vi "Complete_Controller_part_pressures.vi"() -> ()   [LabVIEW 2014]
uses:
  <vilib>/DAQmx/read.llb/DAQmx Read (Analog 1D DBL NChan 1Samp).vi
  <vilib>/DAQmx/write.llb/DAQmx Write (Analog 1D DBL NChan 1Samp).vi
  <vilib>/DAQmx/write.llb/DAQmx Write (Digital Bool 1Line 1Point).vi
  <vilib>/Instr/_visa.llb/VISA Configure Serial Port (Instr).vi
  <vilib>/Utility/file.llb/Read From Spreadsheet File (string).vi
  <vilib>/DAQmx/miscellaneous.llb/DAQmx Fill In Error Info.vi
  Environmental Chamber LabVIEW and Instruments/Drivers and Software/keithley_6430/Keithley 6430/Public/Data/Read (Single Point).vi
  Environmental Chamber LabVIEW and Instruments/Drivers and Software/LabVIEW 8.2 Drivers/keithley_24xx/Keithley 24XX/Public/Data/Read (Single Point).vi
  <vilib>/Utility/file.llb/Write To Spreadsheet File (string).vi
  Environmental Chamber LabVIEW and Instruments/Drivers and Software/keithley_24xx/Keithley 24XX/Keithley 24XX.lvlib
  Environmental Chamber LabVIEW and Instruments/Drivers and Software/keithley_6430/Keithley 6430/Keithley 6430.lvlib
panel:
  in  "Turbo pump\nauto on":bool=TRUE
  in  "Use excel file\nfor sequence?":bool
  out "Sequence time left (hrs)":dbl caption="min"
  out "Sequence Preview":cluster{dbl[], dbl[]}[](graph)
  in  "Import sequence file":path
  out "Chamber relative humidity (%)":dbl
  out "Pressure Control 3":bool caption="Pressure Control"
  in  "valve % open":dbl=100.0 min=0.0 max=100.0 step=5.0
  out "Pressure Control 2":bool caption="Pressure Control"
  out "Keithley 6430":bool
  out "J-Kem":bool caption="J-Kem Temp"
  out "Thermometer":dbl(slide) scale=0.0..150.0
  out "J-Kem Temp (C)":cluster{dbl}(graph)
  out "Keithley 2420":bool caption="Keithley 2430"
  out "Pressure Control":bool
  out "Arduino":bool
  out "SRS QCM":bool
  out "Chamber Pressure (Torr)":cluster{"f":dbl}(graph)
  in  "Start recording after":dbl caption="min"
  in  "Auto stop after":bool
  in  "hrs":dbl=1000.0 min=0.0
  out "Start Time":string
  out "Elapsed (min)":dbl caption="Elapsed Time (s)"
  in  "Delay between data points (s)":dbl caption="sec" min=0.0 max=30.0 format="%#_13g"
  in  "Vapor\nflow\n(sccm)":sgl(slide) min=0 max=100 step=1 scale=0.0..100.0
  out "Actual":dbl
  out "Boolean 3":bool
  out "Actual":dbl
  out "Boolean":bool
  in  "Gas\nflow\n(sccm)":sgl(slide) min=0 max=100 step=1 scale=0.0..100.0
  in  "Turbo pump auto on":bool
  in  "Desired pressure":dbl min=0.0 max=760.0 step=5.0
  out "Valve position (%)":dbl
  in  "Pressure Control":enum32{"Open Mode (%)", "Pressure Mode (Torr)"}(radio)
  in  "stop":bool
  in  "Experiment Notes":string
  in  "Clear all charts":bool
  out "Save data file path":path
  out "Waveform Chart 2":cluster{"f":dbl, "f":dbl}(graph)
  out "Keithley 2420 (Ohm)":cluster{"Resistance":sgl}(graph)
  out "Keithley 6430 (Ohm)":cluster{"Measurement":dbl}(graph)
  out "temp\n(C)":string
  out "gas\nsensor":string
  out "Arduino humidity (%)":cluster{dbl}(graph)
  out "MHz":dbl format="%.6f"
  out "Ohm":dbl format="%.4e"
  out "Waveform Chart 7":cluster{dbl, "Resistance out":dbl}(graph)
  in  "Tab Control":enum32{"Run Sequence", "Create Sequence"}(tab)
  out "User-defined\nsequence 2":string[][](table) caption="Sequence to run"
  in  "Run Sequence":bool
  out "Current step":i32
  out "Step time remaining (min)":dbl caption="min"
  in  "User-defined\nsequence":string[][](table) caption="Create sequence"
  out "QCM mass deposited (g)":cluster{dbl}(graph)
  in  "rapidox O2 Sensor":bool
  in  "setnag O2 Pump":bool
  in  "Baud Rate 2":i32(ring)=2 items=["2400", "4800", "9600", "19200", "38400", "57600", "115200"]
  in  "Com Port":i32(ring) items=["Com 1", "Com 2", "Com 3", "Com 4", "Com 5", "Com 6", "COM 7", "COM 8", "COM 9", "COM 10", "COM 11", "COM 12", "com 13", "COM 14"]
  in  "Com Port 2":i32(ring) items=["Com 1", "Com 2", "Com 3", "Com 4", "Com 5", "Com 6", "COM 7", "COM 8", "COM 9", "COM 10", "COM 11", "COM 12", "com 13", "COM 14"]
  out "Torr":dbl
  out "%":dbl
  out "atm":dbl
  out "Waveform Chart":cluster{dbl}(graph)
  out "O2 Concentration (PPM)":dbl
  out "Waveform Chart 6":cluster{dbl}(graph)
  # "Sample\ntemp (C)"
  # "Currently Unused"
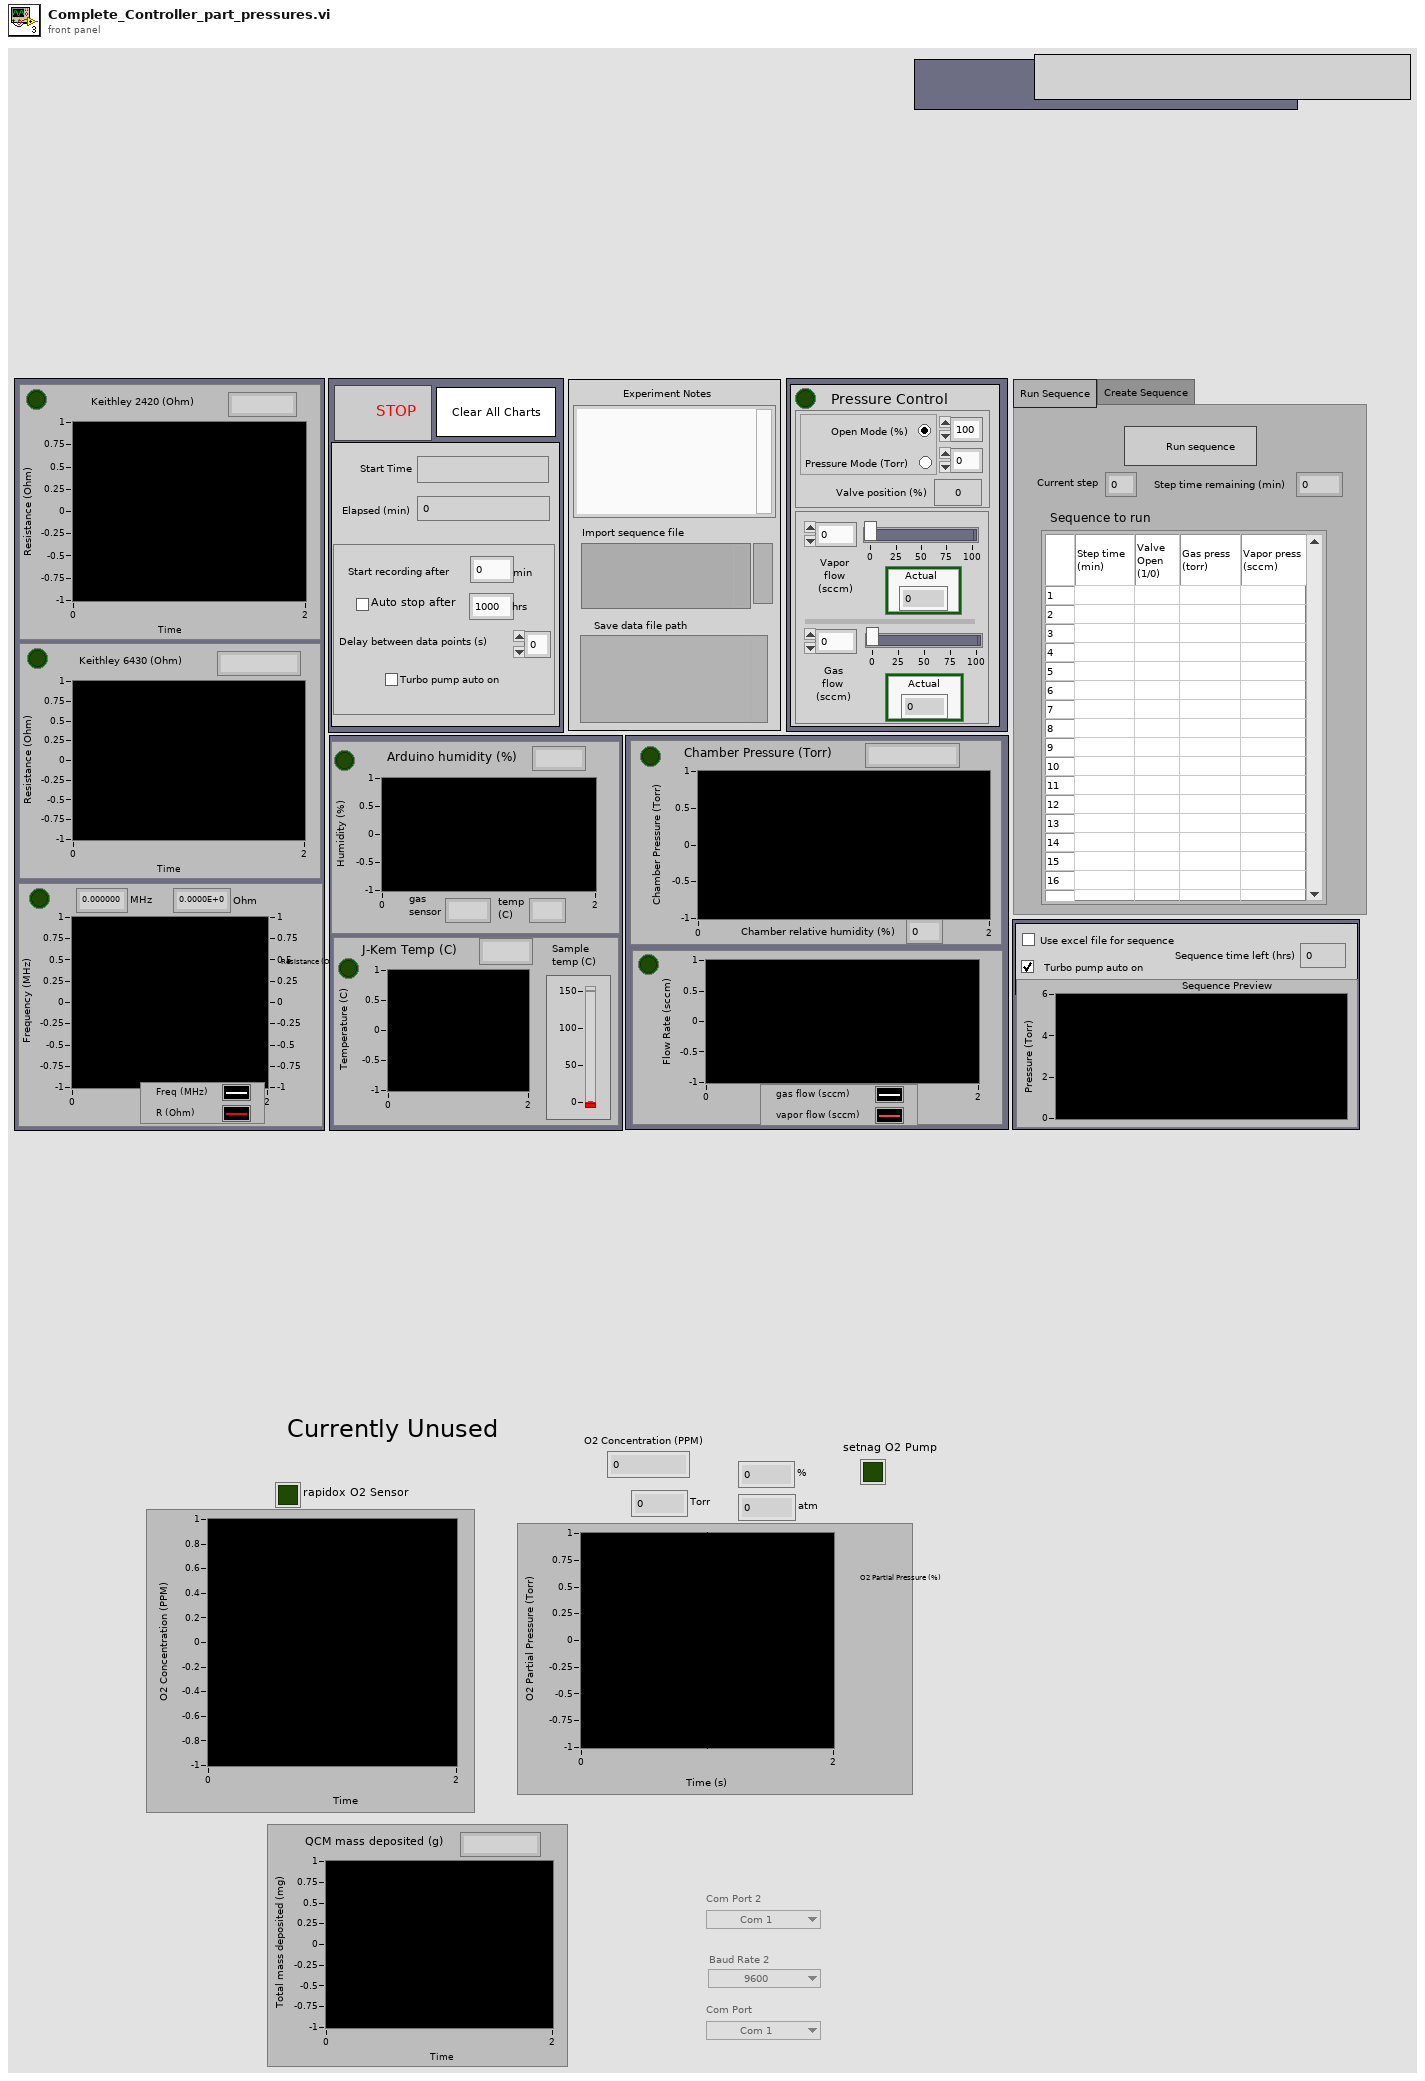
[diagram p1: front panel]
types:
  T1 = enum16{"open", "open or create", "create or replace", "create", "open (read only)"}
  T2 = enum16{"no parity", "odd parity", "even parity", "mark parity", "space parity"}
  T3 = cluster{bool, "VISA resource name":refnum<visa-resource-name>, "error out":errorcluster}
  T4 = cluster{bool, "VISA resource name out":refnum<visa-resource-name>, "error out":errorcluster}
  T5 = cluster{"task out":refnum<k21>, "error out":errorcluster, "task out":refnum<k21>, "error out":errorcluster, "task out":refnum<k21>, "error out":errorcluster, "VISA resource name":refnum<visa-resource-name>, "error out":errorcluster}
  T6 = cluster{"task out":refnum<k21>, "error out":errorcluster, "task out":refnum<k21>, "error out":errorcluster, "task out":refnum<k21>, "error out":errorcluster, "VISA resource name out":refnum<visa-resource-name>, "error out":errorcluster}
  T7 = cluster{bool, "VISA out":refnum<visa-resource-name>, "error out":errorcluster}
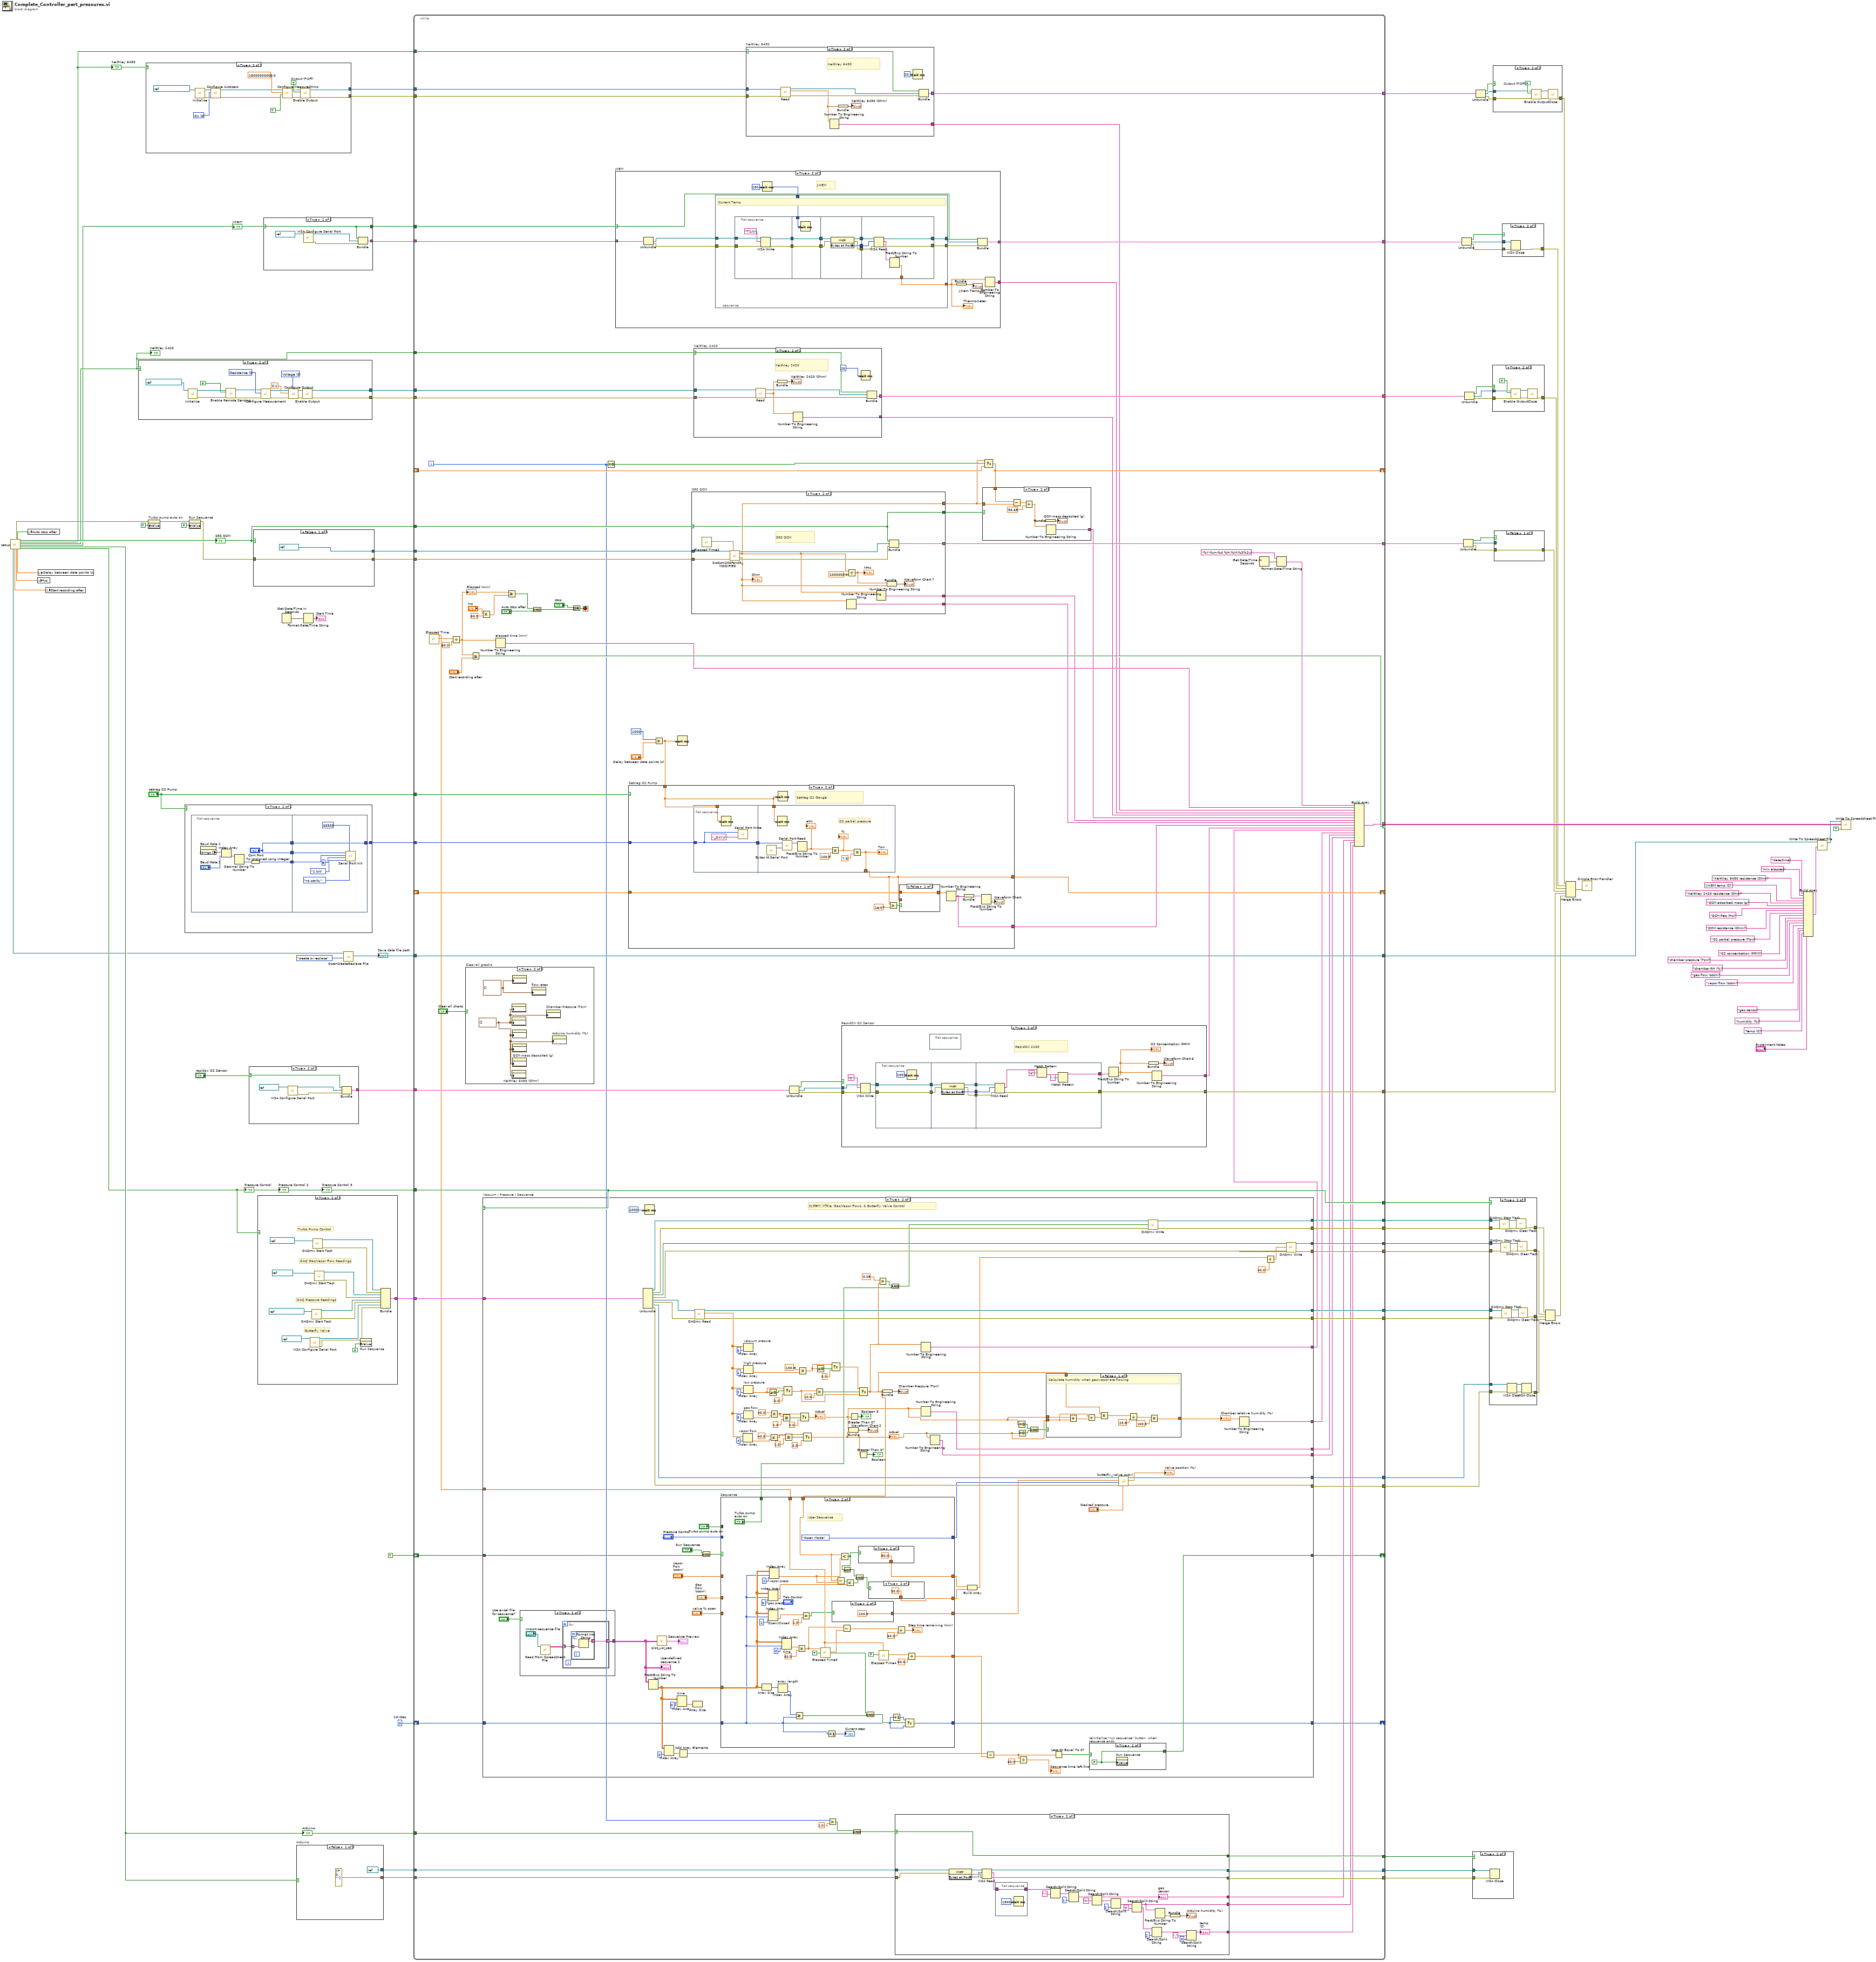
[diagram p0: block diagram]
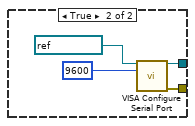
[diagram p3: hidden frame]
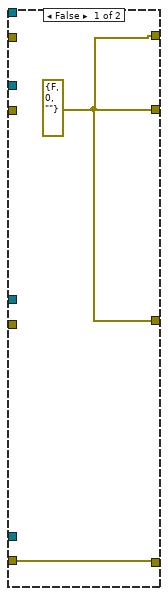
[diagram p4: hidden frame]
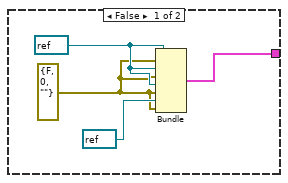
[diagram p5: hidden frame]
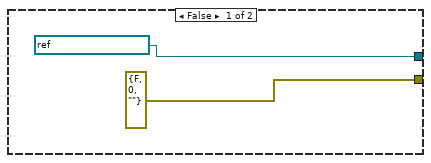
[diagram p7: hidden frame]
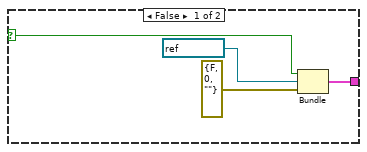
[diagram p8: hidden frame]
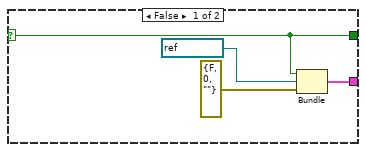
[diagram p10: hidden frame]
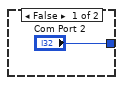
[diagram p11: hidden frame]
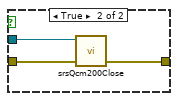
[diagram p12: hidden frame]
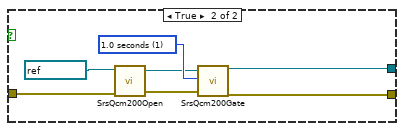
[diagram p13: hidden frame]
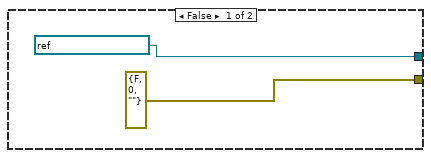
[diagram p15: hidden frame]
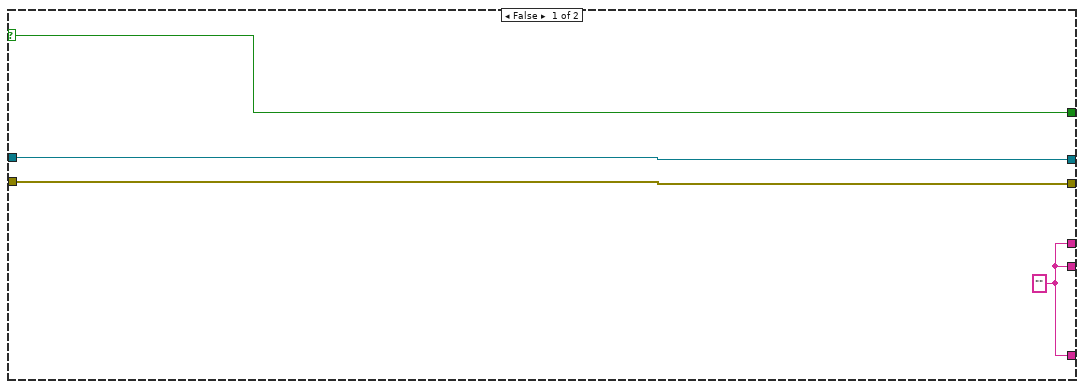
[diagram p16: hidden frame]
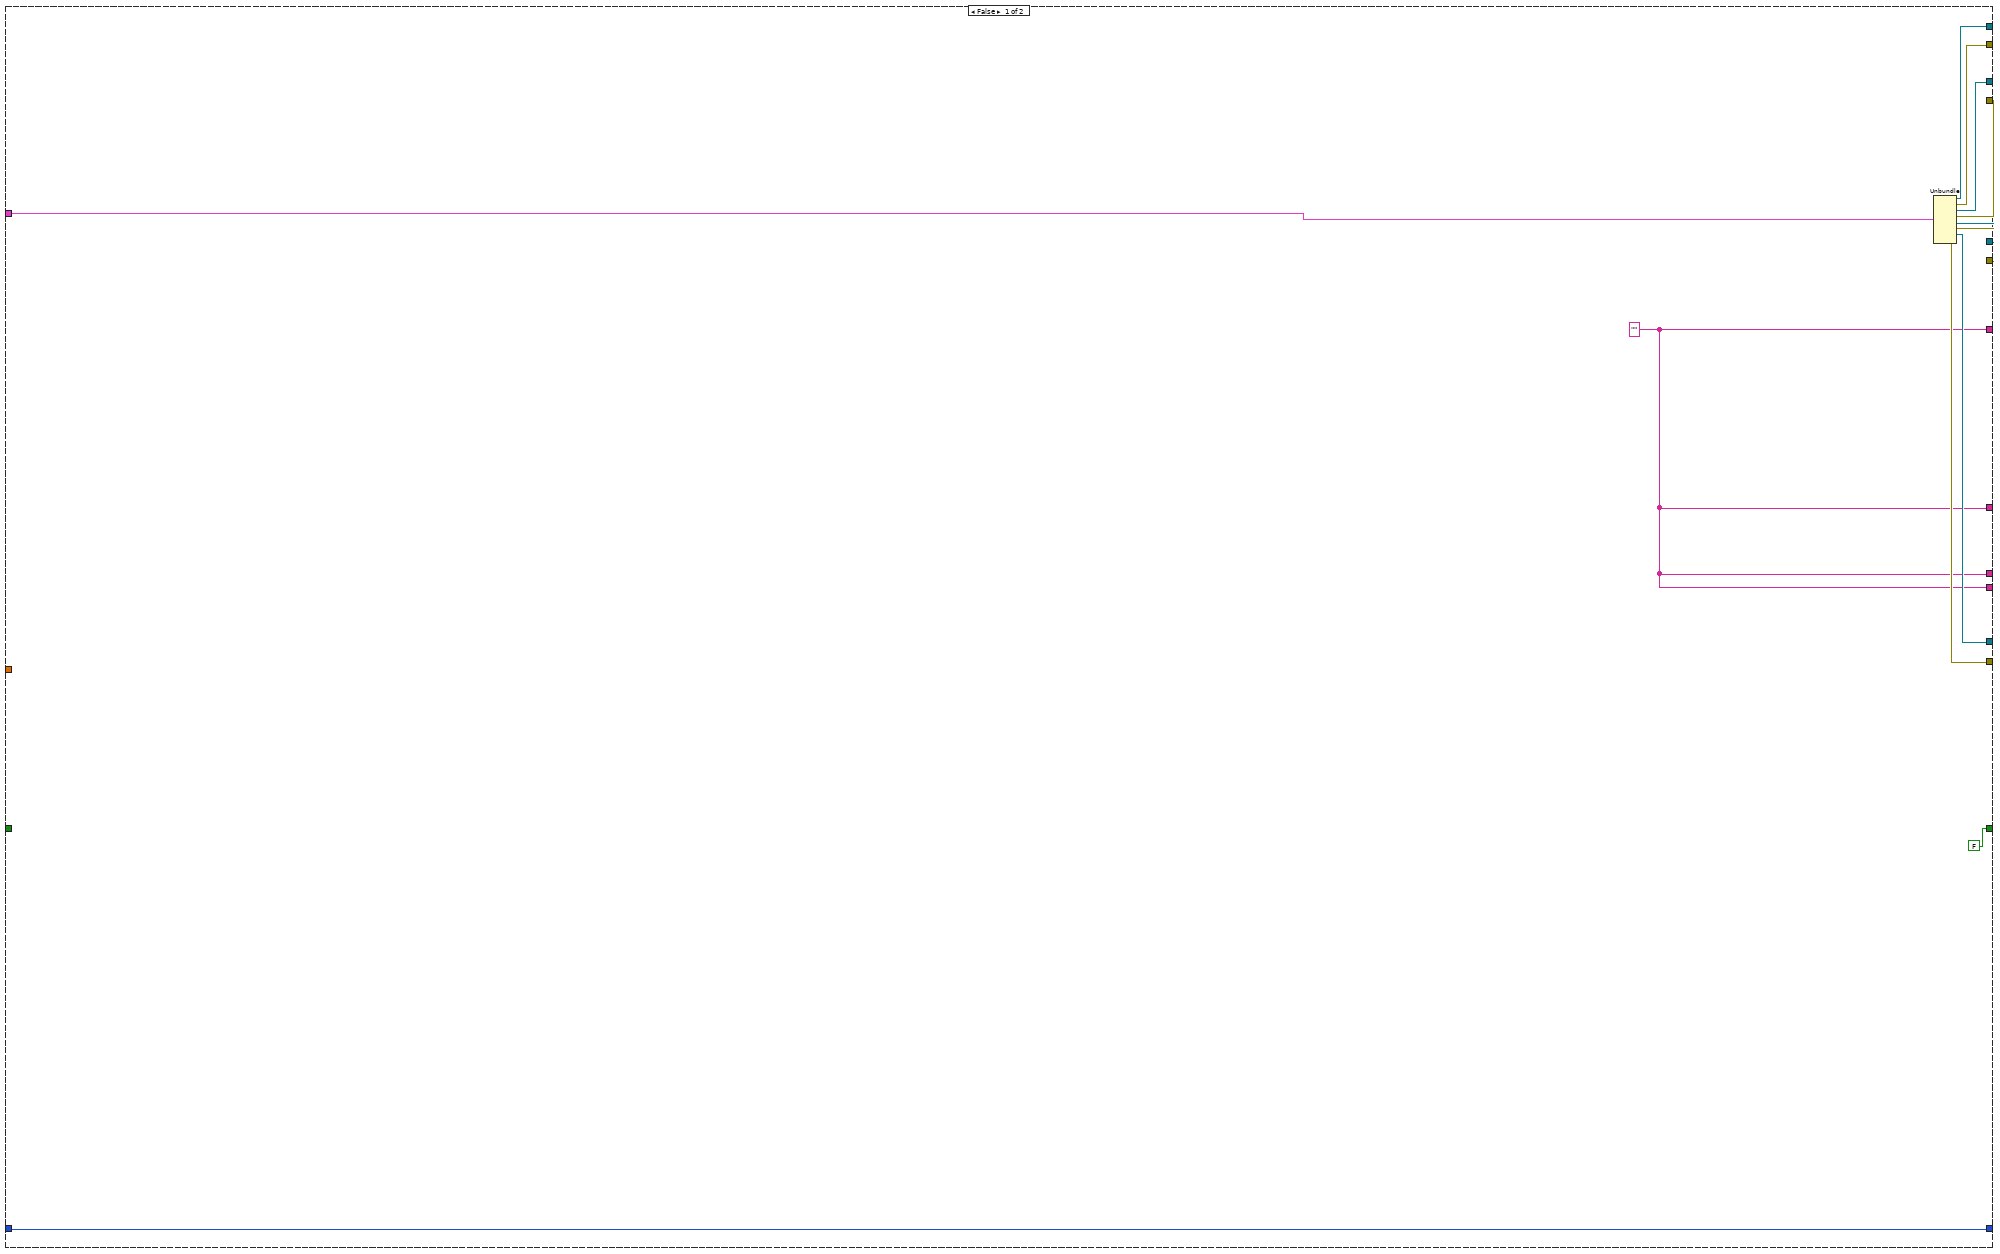
[diagram p17: hidden frame]
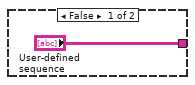
[diagram p18: hidden frame]
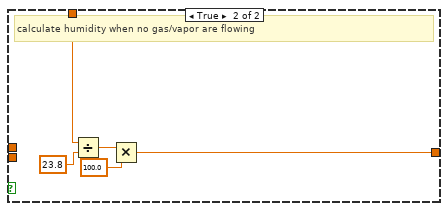
[diagram p19: hidden frame]
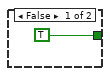
[diagram p20: hidden frame]
diagram:
  w29 = 0  # 1st step
  n1 = call "setup.vi"() -> ("Save file path 2"=w10:path, "begin recording"=w16:dbl, "error IO"=w3:errorcluster, "stop after"=w18:dbl, "Auto Stop 2"=w19:bool, "delay 5"=w17:dbl, "SRS QCM 2"=w15:bool, "Keithley 6431"=w11:bool, "Keithley 2421"=w14:bool, "J-KEM2"=w13:bool, "Arduino2"=w12:bool, "Pressure control 2"=w9:bool)  [unwired: 8 in]
  "SRS QCM" <- w15
  "Arduino" <- w12
  "Pressure Control" <- w9
  "Keithley 2420" <- w14
  "J-Kem" <- w13
  "Keithley 6430" <- w11
  "Pressure Control 2" <- w9
  "Pressure Control 3" <- w9
  n2 = local write "Auto stop after"(w19) -> ()
  n3 = local write "hrs"(w18) -> ()
  n4 = local write "Delay between data points (s)"(w17) -> ()
  n5 = local write "Start recording after"(w16) -> ()
  n6 = case shown="True" w14 {
    tunnel: [refnum<visa-resource-name> "GPIB1::24::INSTR" ("VISA resource name") w108] -> w96
    tunnel: [errorcluster {"status"=FALSE, "code"=0, "source"=""} ("error out") w103] -> w95
    frame False {
    }
    frame True {
      w110 = u16 0 items=["Voltage", "Current"] ("Source Mode  (0: Voltage)")
      w115 = u16 2 items=["Volts", "Current", "Resistance"] ("Function (0: Volts)")
      n7 = call "Initialize.vi"("VISA resource name"=refnum<visa-resource-name> "GPIB1::24::INSTR") -> ("error out"=w104:errorcluster, "VISA resource name out"=w107:refnum<visa-resource-name>)  [unwired: 9 in]
      n8 = call "Enable Remote Sensing.vi"("error in (no error)"=w104, "Enable Remote Sensing (T: Enable)"=FALSE ("4-wire?"), "VISA resource name"=w107) -> ("error out"=w105:errorcluster, "VISA resource name out"=w106:refnum<visa-resource-name>)  [unwired: 7 in]
      n9 = call "Configure Measurement.vi"("error in (no error)"=w105, "Function (0: Volts)"=w115, "VISA resource name"=w106) -> ("error out"=w114:errorcluster, "VISA resource name out"=w113:refnum<visa-resource-name>)  [unwired: 7 in]
      n10 = call "Configure Output.vi"("Source Mode  (0: Voltage)"=w110, "error in (no error)"=w114, "Output Level (0)"=0.1 ("Applied Voltage (V)"), "VISA resource name"=w113) -> ("error out"=w112:errorcluster, "VISA resource name out"=w111:refnum<visa-resource-name>)  [unwired: 6 in]
      n11 = call "Enable Output.vi"("error in (no error)"=w112, "VISA resource name"=w111) -> ("error out"=w103:errorcluster, "VISA resource name out"=w108:refnum<visa-resource-name>)  [unwired: 8 in]
    }
  }
  n12 = case shown="True" w11 {
    tunnel: [refnum<visa-resource-name> "GPIB0::29::INSTR" ("VISA resource name") w126] -> w53
    tunnel: [errorcluster {"status"=FALSE, "code"=0, "source"=""} ("error out") w127] -> w52
    frame False {
    }
    frame True {
      w122 = u16 0 items=["On", "Off", "Once"] ("Autozero  (0: On)")
      w130 = TRUE  # Output (F:Off)
      n13 = call "Initialize.vi"("VISA resource name"=refnum<visa-resource-name> "GPIB0::29::INSTR") -> ("error out"=w123:errorcluster, "VISA resource name out"=w124:refnum<visa-resource-name>)  [unwired: 4 in, 5 out]
      n14 = call "Configure Autozero.vi"("error in (no error)"=w123, "Autozero  (0: On)"=w122, "VISA resource name"=w124) -> ("error out"=w119:errorcluster, "VISA resource name out"=w120:refnum<visa-resource-name>)  [unwired: 7 in]
      n15 = call "Configure MeasureOhms.vi"("error in (no error)"=w119, "Auto Range (T:Enable)"=TRUE, "Resistance Range [Ohms]"=15000000000.0, "VISA resource name"=w120) -> ("error out"=w131:errorcluster, "VISA resource name out"=w129:refnum<visa-resource-name>)  [unwired: 2 in, 4 out]
      n16 = call "Enable Output.vi"("error in (no error)"=w131, "Enable Output (F:Off)"=w130, "VISA resource name"=w129) -> ("error out"=w127:errorcluster, "VISA resource name out"=w126:refnum<visa-resource-name>)  [unwired: 7 out]
    }
  }
  n17 = property on="Turbo pump auto on" class="Bool (strict)"(error in=w3, "Value"=TRUE ("Turbo\npump")) -> (error out=w2:errorcluster)  [unwired: 1 in, 1 out]
  n18 = case shown="True" "setnag O2 Pump" {
    tunnel: ["Com Port 2" w133] -> w92
    frame False {
    }
    frame True {
      n19 = flat-sequence {
        tunnel: ["Com Port"] -> w136
        tunnel: [w138] -> w135
        tunnel: ["Com Port"] -> w134
        tunnel: w136 -> [w144]
        tunnel: w135 -> [w143]
        tunnel: w134 -> [w145]
        tunnel: [w145] -> w133
        frame #0 {
          n20 = property on="Baud Rate 2" class="Ring (strict)"() -> ("Strings []"=w140:string[])  [unwired: 2 in, 2 out]
          n21 = Index Array(array=w140, index="Baud Rate 2") -> (element=w141:string)
          n22 = Decimal String To Number(string=w141) -> (number=w139:i32)  [unwired: 2 in, 1 out]
          n23 = To Unsigned Long Integer(number=w139) -> (unsigned 32bit integer=w138:u32)
        }
        frame #1 {
          n24 = call <vilib>:"Serial Port Init.vi"("parity"=T2."no parity", "buffer size"=u16 65535, "stop bits"=enum16{"1 bit", "1.5 bits", "2 bits"}."1 bit", "data bits"=u16 8, "baud rate"=w143, "port number"=w144) -> ()  [unwired: 1 in, 1 out]
        }
      }
    }
  }
  n25 = property on="Run Sequence" class="Bool (strict)"(error in=w2, "Value"=FALSE ("Run Sequence")) -> (error out=w7:errorcluster)  [unwired: 1 in, 1 out]
  n26 = case shown="True" "rapidox O2 Sensor" {
    selector: "rapidox O2 Sensor" -> [w150 w155]
    tunnel: [w151 w156] -> w63
    frame False {
      n27 = Bundle(w150, "VISA resource name"=refnum<visa-resource-name> "COM7", "error out"=errorcluster {"status"=FALSE, "code"=0, "source"=""}) -> (w151:T3)  [unwired: 1 in]
    }
    frame True {
      n28 = call-poly "VISA Configure Serial Port"("VISA resource name"=refnum<visa-resource-name> "COM7") -> ("VISA resource name out"=w157:refnum<visa-resource-name>, "error out"=w154:errorcluster)  [unwired: 13 in]
      n29 = Bundle(w155, "VISA resource name out"=w157, "error out"=w154) -> (w156:T4)  [unwired: 1 in]
    }
  }
  n30 = case shown="False" w15 {
    tunnel: [refnum<visa-resource-name> "COM6" ("VISA in") w163] -> w94
    tunnel: [w159 w162] -> w93
    tunnel: w7 -> [w159 w161]
    frame False {
    }
    frame True {
      w167 = u16 1 items=["0.1 seconds", "1.0 seconds", "10.0 seconds"] ("Gate in")
      n31 = call "SrsQcm200Open.vi"("error in"=w161, "VISA in"=refnum<visa-resource-name> "COM6") -> ("error out"=w164:errorcluster, "VISA out"=w165:refnum<visa-resource-name>)  [unwired: 3 in]
      n32 = call "SrsQcm200Gate.vi"("VISA in"=w165, "Gate in"=w167, "error in (no error)"=w164) -> ("VISA out"=w163:refnum<visa-resource-name>, "error out"=w162:errorcluster)  [unwired: 14 in, 1 out]
    }
  }
  n33 = case shown="True" w9 {
    tunnel: [w168 w175] -> w34
    frame False {
      w170 = refnum<k21> refnum ("task out")
      w169 = errorcluster {"status"=FALSE, "code"=0, "source"=""} ("error out")
      n34 = Bundle("task out"=w170, "error out"=w169, "task out"=w170, "error out"=w169, "task out"=w170, "error out"=w169, "VISA resource name"=refnum<visa-resource-name> refnum, "error out"=w169) -> (w168:T5)  [unwired: 1 in]
    }
    frame True {
      # "Turbo Pump Control"
      # "DAQ Gas/Vapor Flow Readings"
      # "DAQ Pressure Readings"
      # "Butterfly Valve"
      n35 = call-poly "VISA Configure Serial Port"("VISA resource name"=refnum<visa-resource-name> "COM5") -> ("VISA resource name out"=w176:refnum<visa-resource-name>, "error out"=w172:errorcluster)  [unwired: 13 in]
      n36 = call <vilib>:"DAQmx Start Task.vi"("task/channels in"=refnum<k21> "AllDaqReadings") -> ("task out"=w178:refnum<k21>, "error out"=w177:errorcluster)  [unwired: 13 in]
      n37 = call <vilib>:"DAQmx Start Task.vi"("task/channels in"=refnum<k21> "TurboON") -> ("task out"=w182:refnum<k21>, "error out"=w181:errorcluster)  [unwired: 13 in]
      n38 = call <vilib>:"DAQmx Start Task.vi"("task/channels in"=refnum<k21> "Setflow") -> ("task out"=w180:refnum<k21>, "error out"=w179:errorcluster)  [unwired: 13 in]
      n39 = property on="Run Sequence" class="Bool (strict)"(error in=w172, "Value"=FALSE ("Run Sequence")) -> (error out=w174:errorcluster)  [unwired: 1 in, 1 out]
      n40 = Bundle("task out"=w182, "error out"=w181, "task out"=w180, "error out"=w179, "task out"=w178, "error out"=w177, "VISA resource name out"=w176, "error out"=w174) -> (w175:T6)  [unwired: 1 in]
    }
  }
  n41 = case shown="True" w13 {
    selector: w13 -> [w187 w192]
    tunnel: [w188 w193] -> w81
    tunnel: [w187 w192] -> w75
    frame False {
      n42 = Bundle(w187, "VISA resource name"=refnum<visa-resource-name> "COM3", "error out"=errorcluster {"status"=FALSE, "code"=0, "source"=""}) -> (w188:T3)  [unwired: 1 in]
    }
    frame True {
      n43 = call-poly "VISA Configure Serial Port"("VISA resource name"=refnum<visa-resource-name> "COM3") -> ("VISA resource name out"=w194:refnum<visa-resource-name>, "error out"=w191:errorcluster)  [unwired: 13 in]
      n44 = Bundle(w192, "VISA resource name out"=w194, "error out"=w191) -> (w193:T4)  [unwired: 1 in]
    }
  }
  n45 = Get Date/Time In Seconds() -> (seconds since 1Jan1904=w99:timestamp)
  n46 = case "Arduino" shown="False" w12 {
    tunnel: [refnum<visa-resource-name> refnum ("VISA resource name out") w201] -> w28
    tunnel: [errorcluster {"status"=FALSE, "code"=0, "source"=""} ("error out") w198] -> w27
    frame False {
    }
    frame True {
      n47 = call-poly "VISA Configure Serial Port"("VISA resource name"=refnum<visa-resource-name> "COM12", "baud rate (9600)"=u32 9600) -> ("VISA resource name out"=w201:refnum<visa-resource-name>, "error out"=w198:errorcluster)  [unwired: 12 in]
    }
  }
  n48 = Format Date/Time String(seconds (now)=w99) -> (date/time string=→"Start Time":string)  [unwired: 2 in]
  n49 = call "OpenCreateReplace File.vi"("function (open:0)"=T1."create or replace", "file path"=w10) -> ("new file path"=w20:path)  [unwired: 6 in, 3 out]
  "Save data file path" <- w20
  n50 = while {
    shift-right: [w291] -> _
    shift-left: _ -> [w290]
    tunnel: [w220] -> w97 mode=indexing if=w219
    tunnel: w14 -> [w259]
    tunnel: w96 -> [w288]
    tunnel: w95 -> [w287]
    tunnel: w94 -> [w286]
    tunnel: w93 -> [w285]
    tunnel: w15 -> [w283]
    tunnel: "setnag O2 Pump" -> [w276]
    tunnel: w92 -> [w282]
    tunnel: [w278] -> w89
    tunnel: [w277] -> w85
    tunnel: w81 -> [w275]
    tunnel: [w274] -> w80
    tunnel: w75 -> [w272]
    tunnel: w63 -> [w268]
    tunnel: [w263] -> w61
    tunnel: [w258] -> w60
    tunnel: w20 -> [w258]
    shift-right: [w241] -> _
    shift-left: _ -> [w243]
    tunnel: w53 -> [w255]
    tunnel: w52 -> [w254]
    tunnel: [w253] -> w51
    tunnel: w11 -> [w252]
    tunnel: w9 -> [w233]
    tunnel: [w249] -> w47
    tunnel: [w248] -> w44
    tunnel: [w247] -> w46
    tunnel: [w246] -> w45
    tunnel: [w233] -> w43
    tunnel: [w245] -> w38
    tunnel: w34 -> [w237]
    tunnel: [w236] -> w32
    tunnel: [w235] -> w31
    tunnel: [w234] -> w30
    shift-right: [w232] -> _
    shift-left: w29 -> [w231]
    tunnel: w12 -> [w216]
    tunnel: w28 -> [w226]
    tunnel: w27 -> [w225]
    tunnel: [w224] -> w26
    tunnel: [w223] -> w25
    tunnel: [w222] -> w24
    shift-right: [w207] -> _
    shift-left: TRUE -> [w208]
    i -> [w205]
    stop <- w271 stop-if-true
    n51 = call "Elapsed Time"() -> ("Present (s)"=w230:dbl, "Elapsed Time (s)"=w270:dbl)  [unwired: 12 in, 6 out]
    n52 = Divide(x=w270, y=60.0) -> (x/y=w210:dbl)
    "Elapsed (min)" <- w210
    n53 = case "Clear all graphs" shown="True" "Clear all charts" {
      frame False {
      }
      frame True {
        w547 = cluster{dbl, "Resistance out":dbl}[] [] ("History Data")
        w546 = cluster{dbl}[] [] ("History Data")
        n54 = property on="Keithley 2420 (Ohm)" class="WFChart (strict)"("History Data"=w546) -> ()  [unwired: 2 in, 2 out]
        n55 = property on="J-Kem Temp (C)" class="WFChart (strict)"("History Data"=w546) -> ()  [unwired: 2 in, 2 out]
        n56 = property on="Keithley 6430 (Ohm)" class="WFChart (strict)"("History Data"=w546) -> ()  [unwired: 2 in, 2 out]
        n57 = property on="Waveform Chart 7" class="WFChart (strict)"("History Data"=w547) -> ()  [unwired: 2 in, 2 out]
        n58 = property on="Waveform Chart" class="WFChart (strict)"("History Data"=w546) -> ()  [unwired: 2 in, 2 out]
        n59 = property on="Waveform Chart 6" class="WFChart (strict)"("History Data"=w546) -> ()  [unwired: 2 in, 2 out]
        n60 = property on="QCM mass deposited (g)" class="WFChart (strict)"("History Data"=w546) -> ()  [unwired: 2 in, 2 out]
        n61 = property on="flow rates" class="WFChart (strict)"("History Data"=w547) -> ()  [unwired: 2 in, 2 out]
        n62 = property on="Chamber Pressure (Torr)" class="WFChart (strict)"("History Data"=w546) -> ()  [unwired: 2 in, 2 out]
        n63 = property on="Arduino humidity (%)" class="WFChart (strict)"("History Data"=w546) -> ()  [unwired: 2 in, 2 out]
      }
    }
    n64 = Greater Or Equal?(x=w210, y="Start recording after") -> (x >= y?=w219:bool)
    n65 = Multiply(x="hrs", y=60.0) -> (x*y=w202:dbl)
    n66 = case "Vacuum / Pressure / Sequence" shown="True" w233 {
      tunnel: [w333 w440] -> w248
      tunnel: [w334 w439] -> w246
      tunnel: [w336 w420] -> w249
      tunnel: [w335 w421] -> w247
      tunnel: [w334 w411] -> w245
      tunnel: [w329 w401] -> w240
      tunnel: [w329 w400] -> w239
      tunnel: [w329 w398] -> w238
      tunnel: w237 -> [w339 w396]
      tunnel: [w338 w387] -> w236
      tunnel: [w337 w386] -> w235
      tunnel: [w332 w385] -> w234
      tunnel: w231 -> [w331 w368]
      tunnel: [w331 w382] -> w232
      tunnel: w230 -> [_ w381]
      tunnel: w208 -> [_ w361]
      tunnel: [FALSE ("new element/subarray") w356] -> w207
      tunnel: [w329 w355] -> w206
      frame False {
        w329 = ""
        n67 = Unbundle(w339) -> ("task out"=w338:refnum<k21>, "error out"=w337:errorcluster, "task out"=w336:refnum<k21>, "error out"=w335:errorcluster, "task out"=w333:refnum<k21>, "error out"=w334:errorcluster, "VISA resource name out"=w332:refnum<visa-resource-name>)  [unwired: 1 out]
      }
      frame True {
        # "system info"
        # "DAQ Pressure, Gas/Vapor Flows, & Butterfly Valve Control"
        n68 = case shown="True" "Use excel file\nfor sequence?" {
          tunnel: ["User-defined\nsequence" w443] -> w348
          frame False {
          }
          frame True {
            n69 = call-poly <vilib>:"Read From Spreadsheet File.vi"("file path (dialog if empty)"="Import sequence file") -> ("all rows"=w445:string[][])  [unwired: 6 in, 4 out]
            n70 = for {
              tunnel: w445 -> [w447] mode=indexing
              tunnel: [w446] -> w443 mode=indexing
              n71 = for {
                tunnel: w447 -> [w449] mode=indexing
                tunnel: [w448] -> w446 mode=indexing
                n72 = Format Into String(w449) -> (resulting string=w448:string)  [unwired: 3 in, 1 out]
              }
            }
          }
        }
        "User-defined\nsequence 2" <- w348
        n73 = Unbundle(w396) -> ("task out"=w389:refnum<k21>, "error out"=w388:errorcluster, "task out"=w390:refnum<k21>, "error out"=w391:errorcluster, "task out"=w392:refnum<k21>, "error out"=w393:errorcluster, "VISA resource name out"=w394:refnum<visa-resource-name>, "error out"=w395:errorcluster)
        n74 = Wait (ms)(milliseconds to wait=u32 1000) -> ()  [unwired: 1 out]
        n75 = Fract/Exp String To Number(string=w348) -> (number=w360:dbl[][])  [unwired: 3 in, 1 out]
        n76 = call "plot_usr_seq.vi"("User-defined sequence"=w348) -> ("Sequence Preview"=→"Sequence Preview":cluster{dbl[], dbl[]}[])
        n77 = Index Array(array=w360, index (col)=0 ("disabled index (col)")) -> (element=w372:dbl[])  [unwired: 1 in]
        n78 = Index Array "time"(array=w360, index (row)=0 ("disabled index (col)")) -> (element=w359:dbl[])  [unwired: 1 in]
        n79 = Add Array Elements(numeric array=w372) -> (sum=w365:dbl)
        n80 = Array Size(array=w359) -> ()  [unwired: 1 out]
        n81 = call-poly <vilib>:"DAQmx Read.vi"("task/channels in"=w392, "error in"=w393) -> ("task out"=w440:refnum<k21>, "data"=w431:dbl[], "error out"=w439:errorcluster)  [unwired: 11 in]
        n82 = And(x="Run Sequence", y=w361) -> (x .and. y?=w362:bool)
        n83 = Index Array "vapor flow"(array=w431, index=4) -> (element=w427:dbl)
        n84 = Index Array "vacuum presure"(array=w431, index=0) -> ()  [unwired: 1 out]
        n85 = Index Array "high pressure"(array=w431, index=1) -> (element=w434:dbl)
        n86 = Index Array "low pressure"(array=w431, index=2) -> (element=w405:dbl)
        n87 = Index Array "gas flow"(array=w431, index=3) -> (element=w429:dbl)
        n88 = Greater Or Equal To 0?(x=w405) -> (x >= 0?=w406:bool)
        n89 = Multiply(x=40.0, y=w427) -> (x*y=w418:dbl)
        n90 = Multiply(x=40.0, y=w429) -> (x*y=w415:dbl)
        n91 = Greater Or Equal?(x=w415, y=1.0) -> (x >= y?=w414:bool)
        n92 = Select(t=w405, s=w406, f=0.0) -> (s? t:f=w404:dbl)
        n93 = Greater Or Equal?(x=w418, y=1.0) -> (x >= y?=w417:bool)
        n94 = Multiply(x=100.0, y=w434) -> (x*y=w422:dbl)
        n95 = Select(t=w415, s=w414, f=0.0) -> (s? t:f=w350:dbl)
        "Actual" <- w350
        n96 = Select(t=w418, s=w417, f=0.0) -> (s? t:f=w349:dbl)
        "Actual" <- w349
        n97 = Greater?(x=w404, y=10.0) -> (0:w410:bool)
        n98 = Greater Or Equal To 0?(x=w422) -> (x >= 0?=w424:bool)
        n99 = Select(t=w422, s=w424, f=0.0) -> (s? t:f=w409:dbl)
        n100 = Bundle("f"=w350, "f"=w349) -> (→"Waveform Chart 2":cluster{"f":dbl, "f":dbl})  [unwired: 1 in]
        n101 = Greater Than 0?(x=w350) -> (x > 0?=→"Boolean 3":bool)
        n102 = Select(t=w409, s=w410, f=w404) -> (s? t:f=w340:dbl)
        n103 = case "Sequence" shown="True" w362 {
          tunnel: w381 -> [_ w502]
          tunnel: [w473 w503] -> w382
          tunnel: w368 -> [w473 w489]
          tunnel: "Vapor\nflow\n(sccm)" -> [w472 _]
          tunnel: "Gas\nflow\n(sccm)" -> [w471 _]
          tunnel: [w472 w483] -> w378
          tunnel: [w471 w474] -> w377
          tunnel: "Turbo pump auto on" -> [w470 _]
          tunnel: [w470 "Turbo pump\nauto on"] -> w374
          tunnel: w360 -> [_ w496]
          tunnel: "Pressure Control" -> [w469 _]
          tunnel: [w469 enum32{"Open Mode", "Pressure Mode"}."Open Mode" ("Pressure Control")] -> w369
          tunnel: [0.0 w499] -> w364
          tunnel: "valve % open" -> [w467 _]
          tunnel: [w467 w484] -> w341
          tunnel: w340 -> [_ w478]
          frame False {
          }
          frame True {
            # "User Sequence"
            n104 = Array Size(array=w496) -> (size(s)=w516:i32[])
            n105 = Index Array "gas press"(array=w496, index (row)=w489, index (col)=3 ("disabled index (col)")) -> (element=w477:dbl)
            n106 = Index Array "Open/Closed"(array=w496, index (row)=w489, index (col)=1 ("disabled index (col)")) -> (element=w487:dbl)
            n107 = Index Array "vapor press"(array=w496, index (row)=w489, index (col)=2 ("disabled index (col)")) -> (element=w476:dbl)
            n108 = Index Array "array length"(array=w516) -> (element=w497:i32)  [unwired: 1 in]
            n109 = Index Array "time"(array=w496, index (row)=w489, index (col)=0) -> (element=w508:dbl)
            n110 = Greater Or Equal?(x=w497, y=w489) -> (x >= y?=w513:bool)
            n111 = Multiply(x=w508, y=60.0) -> (x*y=w494:dbl)
            n112 = Equal?(x=w487, y=1.0) -> (x = y?=w485:bool)
            n113 = call "Elapsed Time3"("Time Target (s)"=w494, "Auto Reset"=TRUE, "Set Start Time (s)"=w502) -> ("Elapsed Time (s)"=w493:dbl, "Time has Elapsed"=w512:bool)  [unwired: 9 in, 6 out]
            n114 = Increment(x=w489) -> (x+1=→"Current step":i32)
            n115 = case shown="True" w485 {
              tunnel: [0.0 100.0] -> w484
              frame False {
              }
              frame True {
              }
            }
            n116 = Subtract(x=w478, y=w476) -> (x-y=w479:dbl)
            n117 = Less?(x=w478, y=w476) -> (x < y?=w482:bool)
            n118 = Subtract(x=w494, y=w493) -> (x-y=w490:dbl)
            n119 = Not(x=w482) -> (.not. x?=w481:bool)
            n120 = Less?(x=w479, y=w477) -> (x < y?=w480:bool)
            n121 = And(x=w481, y=w480) -> (x .and. y?=w475:bool)
            n122 = case shown="True" w482 {
              tunnel: [0.0 50.0] -> w483
              frame False {
              }
              frame True {
              }
            }
            n123 = And(x=w512, y=w513) -> (x .and. y?=w505:bool)
            n124 = case shown="True" w475 {
              tunnel: [0.0 50.0] -> w474
              frame False {
              }
              frame True {
              }
            }
            n125 = call "Elapsed Time4"("Reset"=FALSE, "Set Start Time (s)"=w502) -> ("Elapsed Time (s)"=w500:dbl)  [unwired: 10 in, 7 out]
            n126 = Increment(x=w489) -> (x+1=w504:i32)
            n127 = Divide(x=w490, y=60.0) -> (x/y=→"Step time remaining (min)":dbl)
            n128 = Select(t=w504, s=w505, f=w489) -> (s? t:f=w503:i32)
            n129 = Divide(x=w500, y=60.0) -> (x/y=w499:dbl)
          }
        }
        n130 = Greater Than 0?(x=w349) -> (x > 0?=→"Boolean":bool)
        n131 = Greater?(x=0.05, y=w340) -> (0:w373:bool)
        n132 = Bundle("f"=w340) -> (→"Chamber Pressure (Torr)":cluster{"f":dbl})  [unwired: 1 in]
        n133 = And(x=w373, y=w374) -> (x .and. y?=w383:bool)
        n134 = Number To Engineering String(4:w350) -> (0:w400:string)  [unwired: 3 in]
        n135 = Number To Engineering String(4:w340) -> (0:w401:string)  [unwired: 3 in]
        n136 = Number To Engineering String(4:w349) -> (0:w398:string)  [unwired: 3 in]
        n137 = Build Array(w378, w377) -> (w376:dbl[])
        n138 = Subtract(x=w365, y=w364) -> (x-y=w345:dbl)
        n139 = Equal To 0?(x=w350) -> (x = 0?=w353:bool)
        n140 = Equal To 0?(x=w349) -> (x = 0?=w354:bool)
        n141 = Divide(x=w345, y=60.0) -> (x/y=→"Sequence time left (hrs)":dbl)
        n142 = And(x=w353, y=w354) -> (x .and. y?=w352:bool)
        n143 = case shown="False" w352 {
          tunnel: w340 -> [w451 w461]
          tunnel: [w450 w460] -> w351
          tunnel: w350 -> [w459 _]
          tunnel: w349 -> [w457 _]
          frame False {
            # "Calculate humidity when gas/vapor are flowing"
            n144 = Add(x=w459, y=w457) -> (x+y=w458:dbl)
            n145 = Divide(x=w457, y=w458) -> (x/y=w452:dbl)
            n146 = Multiply(x=w451, y=w452) -> (x*y=w453:dbl)
            n147 = Divide(x=w453, y=23.8) -> (x/y=w455:dbl)
            n148 = Multiply(x=w455, y=100.0) -> (x*y=w450:dbl)
          }
          frame True {
            # "calculate humidity when no gas/vapor are flowing"
            n149 = Divide(x=w461, y=23.8) -> (x/y=w463:dbl)
            n150 = Multiply(x=w463, y=100.0) -> (x*y=w460:dbl)
          }
        }
        "Chamber relative humidity (%)" <- w351
        n151 = Less Or Equal To 0?(x=w345) -> (x <= 0?=w357:bool)
        n152 = case "reinitialize \"run sequence\" button  when sequence ends" shown="True" w357 {
          tunnel: [TRUE ("Run Sequence") w466] -> w356
          frame False {
          }
          frame True {
            w466 = FALSE ("Run Sequence")
            n153 = property on="Run Sequence" class="Bool (strict)"("Value"=w466) -> ()  [unwired: 2 in, 2 out]
          }
        }
        n154 = call "butterfly_valve_subvi.vi"("Desired pressure"="Desired pressure", "error in (no error)"=w395, "Pressure Control"=w369, 10:w341, "VISA Refnum in"=w394) -> ("error out"=w411:errorcluster, "Valve position (%)"=→"Valve position (%)":dbl, "VISA Refnum out"=w385:refnum<visa-resource-name>)  [unwired: 4 in]
        n155 = call-poly <vilib>:"DAQmx Write.vi"("task/channels in"=w389, "data"=w383, "error in"=w388) -> ("task out"=w387:refnum<k21>, "error out"=w386:errorcluster)  [unwired: 10 in, 1 out]
        n156 = Number To Engineering String(4:w351) -> (0:w355:string)  [unwired: 3 in]
        n157 = Divide(x=w376, y=40.0 ("Waveform")) -> (x/y=w413:dbl[])
        n158 = call-poly <vilib>:"DAQmx Write.vi"("task/channels in"=w390, "data"=w413, "error in"=w391) -> ("task out"=w420:refnum<k21>, "error out"=w421:errorcluster)  [unwired: 10 in, 1 out]
      }
    }
    n159 = Number To Engineering String "elapsed time (min)"(4:w210) -> (0:w292:string)  [unwired: 3 in]
    n160 = Greater Or Equal?(x=w210, y=w202) -> (x >= y?=w213:bool)
    n161 = And(x=w213, y="Auto stop after") -> (x .and. y?=w211:bool)
    n162 = Or(x="stop", y=w211) -> (x .or. y?=w271:bool)
    n163 = Equal To 0?(x=w205) -> (x = 0?=w244:bool)
    n164 = case "JKEM" shown="True" w272 {
      selector: w272 -> [_ w585]
      tunnel: w275 -> [w583 w590]
      tunnel: [w583 w588] -> w274
      tunnel: ["" w586] -> w273
      frame False {
      }
      frame True {
        w594 = u32 150 ("milliseconds to wait")
        # "J-KEM"
        n165 = Unbundle(w590) -> ("VISA resource name out"=w589:refnum<visa-resource-name>, "error out"=w584:errorcluster)  [unwired: 1 out]
        n166 = stacked-sequence {
          tunnel: w589 -> [w600]
          tunnel: w584 -> [w599]
          tunnel: w594 -> [w598]
          tunnel: [w596] -> w591
          tunnel: [w595] -> w592
          tunnel: [w597] -> w587
          frame #0 {
            # "Current Temp"
            n167 = flat-sequence {
              tunnel: w600 -> [w612]
              tunnel: w599 -> [w611]
              tunnel: [w609] -> w607
              tunnel: [w608] -> w606
              tunnel: w598 -> [w615]
              tunnel: [w614] -> w605
              tunnel: w607 -> [w614]
              tunnel: w606 -> [w613]
              tunnel: [w613] -> w604
              tunnel: w605 -> [w620]
              tunnel: w604 -> [w619]
              tunnel: [w618] -> w603
              tunnel: [w617] -> w602
              tunnel: [w616] -> w601
              tunnel: w603 -> [w627]
              tunnel: w602 -> [w626]
              tunnel: w601 -> [w625]
              tunnel: [w622] -> w595
              tunnel: [w623] -> w596
              tunnel: [w621] -> w597
              frame #0 {
                n168 = VISA Write(VISA resource name=w612, write buffer="T(1)\r", error in (no error)=w611) -> (VISA resource name out=w609:refnum<visa-resource-name>, error out=w608:errorcluster)  [unwired: 1 out]
              }
              frame #1 {
                n169 = Wait (ms)(milliseconds to wait=w615) -> ()  [unwired: 1 out]
              }
              frame #2 {
                n170 = property class="Instr"(reference=w620, error in=w619) -> (reference out=w618:refnum<visa-resource-name>, error out=w616:errorcluster, "Bytes at Port"=w617:u32)
              }
              frame #3 {
                n171 = VISA Read(VISA resource name=w627, byte count=w626, error in (no error)=w625) -> (VISA resource name out=w623:refnum<visa-resource-name>, read buffer=w624:string, error out=w622:errorcluster)  [unwired: 1 out]
                n172 = Fract/Exp String To Number(string=w624) -> (number=w621:dbl)  [unwired: 3 in, 1 out]
              }
            }
          }
        }
        "Thermometer" <- w587
        n173 = Wait (ms)(milliseconds to wait=w594) -> ()  [unwired: 1 out]
        n174 = Bundle(w587) -> (→"J-Kem Temp (C)":cluster{dbl})  [unwired: 1 in]
        n175 = Bundle(w585, "VISA resource name out"=w591, "error out"=w592) -> (w588:T4)  [unwired: 1 in]
        n176 = Number To Engineering String(4:w587) -> (0:w586:string)  [unwired: 3 in]
      }
    }
    n177 = Multiply(x=u32 1000, y="Delay between data points (s)") -> (x*y=w262:dbl)
    n178 = case "Setnag O2 Pump" shown="True" w276 {
      tunnel: [w664 w668] -> w291
      tunnel: w290 -> [w664 w669]
      tunnel: w262 -> [_ w665]
      tunnel: w282 -> [_ w667]
      tunnel: ["" w666] -> w281
      frame False {
      }
      frame True {
        # "SetNag O2 Gauge"
        n179 = flat-sequence {
          tunnel: [w678] -> w675
          tunnel: w665 -> [w680]
          tunnel: w667 -> [w678]
          tunnel: w675 -> [w681]
          tunnel: w665 -> [w688]
          tunnel: [w684] -> w668
          frame #0 {
            n180 = Wait (ms)(milliseconds to wait=w680) -> ()  [unwired: 1 out]
            n181 = call <vilib>:"Serial Port Write.vi"("string to write"="_OXY\r" ("O2 partial press"), "port number"=w678) -> ()  [unwired: 1 out]
          }
          frame #1 {
            # "O2 partial pressure"
            n182 = call <vilib>:"Bytes At Serial Port.vi"() -> ("byte count"=w689:u32)  [unwired: 1 in, 1 out]
            n183 = Wait (ms)(milliseconds to wait=w688) -> ()  [unwired: 1 out]
            n184 = call <vilib>:"Serial Port Read.vi"("requested byte count"=w689, "port number"=w681) -> ("string read"=w687:string)  [unwired: 1 out]
            n185 = Fract/Exp String To Number(string=w687) -> (number=w685:dbl)  [unwired: 3 in, 1 out]
            "atm" <- w685
            n186 = Multiply(x=w685, y=100.0) -> (x*y=w682:dbl)
            "%" <- w682
            n187 = Multiply(x=w682, y=7.6) -> (x*y=w684:dbl)
            "Torr" <- w684
          }
        }
        n188 = Wait (ms)(milliseconds to wait=w665) -> ()  [unwired: 1 out]
        n189 = Greater?(x=w668, y=1e-07) -> (0:w671:bool)
        n190 = case shown="False" w671 {
          tunnel: [w676 w677] -> w670
          tunnel: w668 -> [_ w677]
          tunnel: w669 -> [w676 _]
          frame False {
          }
          frame True {
          }
        }
        n191 = Number To Engineering String(4:w670) -> (0:w666:string)  [unwired: 3 in]
        n192 = Bundle(w666) -> (w673:cluster{string})  [unwired: 1 in]
        n193 = Fract/Exp String To Number(string=w673) -> (number=→"Waveform Chart":cluster{dbl})  [unwired: 3 in, 1 out]
      }
    }
    n194 = Wait (ms)(milliseconds to wait=w262) -> ()  [unwired: 1 out]
    n195 = case "SRS QCM" shown="True" w283 {
      selector: w283 -> [w643 w649]
      tunnel: w286 -> [w647 w655]
      tunnel: w285 -> [w646 w657]
      tunnel: [w648 w662] -> w284
      tunnel: [w648 w661] -> w280
      tunnel: [w645 w660] -> w277
      tunnel: [0.0 w650] -> w242
      tunnel: [w643 w649] -> w250
      frame False {
        w648 = ""
        n196 = Bundle(w643, "VISA out"=w647, "error out"=w646) -> (w645:T7)  [unwired: 1 in]
      }
      frame True {
        # "SRS QCM"
        n197 = call "Elapsed Time2"() -> ("Elapsed Time (s)"=w656:dbl)  [unwired: 12 in, 7 out]
        n198 = call "SrsQcm200FandR_MODIFIED.vi"("VISA in"=w655, "Reference time in"=w656, "error in (no error)"=w657) -> ("VISA out"=w653:refnum<visa-resource-name>, "Frequency out"=w650:dbl, "Resistance out"=w652:dbl, "error out"=w654:errorcluster)  [unwired: 6 in, 3 out]
        "Ohm" <- w652
        n199 = Number To Engineering String(4:w652) -> (0:w661:string)  [unwired: 3 in]
        n200 = Divide(x=w650, y=1000000.0) -> (x/y=w651:dbl)
        "MHz" <- w651
        n201 = Number To Engineering String(4:w650) -> (0:w662:string)  [unwired: 3 in]
        n202 = Bundle(w651, "Resistance out"=w652) -> (→"Waveform Chart 7":cluster{dbl, "Resistance out":dbl})  [unwired: 1 in]
        n203 = Bundle(w649, "VISA out"=w653, "error out"=w654) -> (w660:T7)  [unwired: 1 in]
      }
    }
    n204 = case "Keithley 2420" shown="True" w259 {
      selector: w259 -> [w631 w639]
      tunnel: w288 -> [w630 w634]
      tunnel: w287 -> [w629 w633]
      tunnel: [w628 w637] -> w278
      tunnel: ["" w636] -> w279
      frame False {
        n205 = Bundle(w631, "VISA resource name out"=w630, "error out"=w629) -> (w628:T4)  [unwired: 1 in]
      }
      frame True {
        # "Keithley 2420"
        n206 = call-poly "Read.vi"("VISA resource name"=w634, "error in (no error)"=w633) -> ("VISA resource name out"=w640:refnum<visa-resource-name>, "Resistance"=w635:sgl, "error out"=w638:errorcluster)  [unwired: 7 in, 4 out]
        n207 = Bundle("Resistance"=w635) -> (→"Keithley 2420 (Ohm)":cluster{"Resistance":sgl})  [unwired: 1 in]
        n208 = Number To Engineering String(4:w635) -> (0:w636:string)  [unwired: 3 in]
        n209 = Wait (ms)(milliseconds to wait=u32 20) -> ()  [unwired: 1 out]
        n210 = Bundle(w639, "VISA resource name out"=w640, "error out"=w638) -> (w637:T4)  [unwired: 1 in]
      }
    }
    n211 = case "Keithley 6430" shown="True" w252 {
      selector: w252 -> [w534 w544]
      tunnel: w255 -> [w533 w541]
      tunnel: w254 -> [w532 w540]
      tunnel: ["" w543] -> w214
      tunnel: [w531 w542] -> w253
      frame False {
        n212 = Bundle(w534, "VISA resource name out"=w533, "error out"=w532) -> (w531:T4)  [unwired: 1 in]
      }
      frame True {
        # "Keithley 6430"
        n213 = call-poly "Read.vi"("error in (no error)"=w540, "VISA resource name"=w541) -> ("error out"=w539:errorcluster, "Measurement"=w537:dbl, "VISA resource name out"=w538:refnum<visa-resource-name>)  [unwired: 1 in, 6 out]
        n214 = Number To Engineering String(4:w537) -> (0:w543:string)  [unwired: 3 in]
        n215 = Bundle("Measurement"=w537) -> (→"Keithley 6430 (Ohm)":cluster{"Measurement":dbl})  [unwired: 1 in]
        n216 = Wait (ms)(milliseconds to wait=u32 20) -> ()  [unwired: 1 out]
        n217 = Bundle(w544, "VISA resource name out"=w538, "error out"=w539) -> (w542:T4)  [unwired: 1 in]
      }
    }
    n218 = Unbundle(w268) -> (w267:bool, "VISA resource name out"=w266:refnum<visa-resource-name>, "error out"=w265:errorcluster)
    n219 = Greater?(x=w205, y=1.0) -> (0:w215:bool)
    n220 = case "RapidOX O2 Sensor" shown="True" w267 {
      tunnel: w266 -> [_ w555]
      tunnel: w265 -> [w548 w554]
      tunnel: ["" w553] -> w264
      tunnel: [w548 w550] -> w263
      frame False {
      }
      frame True {
        # "RapidOX 2100"
        n221 = VISA Write(VISA resource name=w555, write buffer="D", error in (no error)=w554) -> (VISA resource name out=w558:refnum<visa-resource-name>, error out=w557:errorcluster)  [unwired: 1 out]
        n222 = flat-sequence {
          tunnel: [w567] -> w564
          tunnel: [w565] -> w563
          tunnel: w558 -> [w567]
          tunnel: w557 -> [w565]
          tunnel: w564 -> [w572]
          tunnel: w563 -> [w571]
          tunnel: [w570] -> w562
          tunnel: [w569] -> w561
          tunnel: [w568] -> w560
          tunnel: w562 -> [w581]
          tunnel: w561 -> [w580]
          tunnel: w560 -> [w579]
          tunnel: [w578] -> w550
          tunnel: [w573] -> w552
          frame #0 {
            n223 = Wait (ms)(milliseconds to wait=u32 100) -> ()  [unwired: 1 out]
          }
          frame #1 {
            n224 = property class="Instr"(reference=w572, error in=w571) -> (reference out=w570:refnum<visa-resource-name>, error out=w568:errorcluster, "Bytes at Port"=w569:u32)
          }
          frame #2 {
            n225 = VISA Read(VISA resource name=w581, byte count=w580, error in (no error)=w579) -> (read buffer=w576:string, error out=w578:errorcluster)  [unwired: 2 out]
            n226 = Match Pattern(string=w576, regular expression="d") -> (after substring=w574:string)  [unwired: 1 in, 3 out]
            n227 = Match Pattern(string=w574, regular expression=",") -> (before substring=w573:string)  [unwired: 1 in, 3 out]
          }
        }
        n228 = flat-sequence {
          frame #0 {
          }
        }
        n229 = Fract/Exp String To Number(string=w552) -> (number=w551:dbl)  [unwired: 3 in, 1 out]
        "O2 Concentration (PPM)" <- w551
        n230 = Bundle(w551) -> (→"Waveform Chart 6":cluster{dbl})  [unwired: 1 in]
        n231 = Number To Engineering String(4:w551) -> (0:w553:string)  [unwired: 3 in]
      }
    }
    n232 = And(x=w215, y=w216) -> (x .and. y?=w227:bool)
    n233 = case shown="True" w227 {
      selector: w227 -> [w295 w326]
      tunnel: w226 -> [w297 w305]
      tunnel: w225 -> [w296 w306]
      tunnel: [w297 w309] -> w223
      tunnel: [w296 w308] -> w222
      tunnel: [w295 w326] -> w224
      tunnel: [w294 w307] -> w221
      tunnel: [w294 w300] -> w217
      tunnel: [w294 w304] -> w218
      frame False {
        w294 = ""
      }
      frame True {
        n234 = property class="Instr"(reference=w305, error in=w306) -> (reference out=w323:refnum<visa-resource-name>, error out=w325:errorcluster, "Bytes at Port"=w324:u32)
        n235 = VISA Read(VISA resource name=w323, byte count=w324, error in (no error)=w325) -> (VISA resource name out=w309:refnum<visa-resource-name>, read buffer=w298:string, error out=w308:errorcluster)  [unwired: 1 out]
        n236 = flat-sequence {
          tunnel: [w328] -> w299
          tunnel: w298 -> [w328]
          frame #0 {
            n237 = Wait (ms)(milliseconds to wait=u32 1500) -> ()  [unwired: 1 out]
          }
        }
        n238 = Search/Split String(string=w299, search string/char (-)=":") -> (match + rest of string=w320:string)  [unwired: 1 in, 2 out]
        n239 = Search/Split String(string=w320, offset (0)=1) -> (match + rest of string=w318:string)  [unwired: 1 in, 2 out]
        n240 = Search/Split String(string=w318, search string/char (-)="h") -> (substring before match=w307:string, match + rest of string=w316:string)  [unwired: 1 in, 1 out]
        "gas\nsensor" <- w307
        n241 = Search/Split String(string=w316, offset (0)=2) -> (match + rest of string=w314:string)  [unwired: 1 in, 2 out]
        n242 = Search/Split String(string=w314, search string/char (-)="t") -> (substring before match=w304:string, match + rest of string=w312:string)  [unwired: 1 in, 1 out]
        n243 = Search/Split String(string=w312, offset (0)=2) -> (match + rest of string=w302:string)  [unwired: 1 in, 2 out]
        n244 = Fract/Exp String To Number(string=w304) -> (number=w310:dbl)  [unwired: 3 in, 1 out]
        n245 = Bundle(w310) -> (→"Arduino humidity (%)":cluster{dbl})  [unwired: 1 in]
        n246 = Search/Split String(string=w302, search string/char (-)=".", offset (0)=0) -> (substring before match=w300:string)  [unwired: 2 out]
        "temp\n(C)" <- w300
      }
    }
    n247 = Select(t=w242, s=w244, f=w243) -> (s? t:f=w241:dbl)
    n248 = case shown="True" w250 {
      tunnel: w242 -> [_ w528]
      tunnel: ["" w526] -> w256
      tunnel: w241 -> [_ w525]
      frame False {
      }
      frame True {
        n249 = Subtract(x=w525, y=w528) -> (x-y=w529:dbl)
        n250 = Divide(x=w529, y=56.65) -> (x/y=w524:dbl)
        n251 = Bundle(w524) -> (→"QCM mass deposited (g)":cluster{dbl})  [unwired: 1 in]
        n252 = Number To Engineering String(4:w524) -> (0:w526:string)  [unwired: 3 in]
      }
    }
    n253 = Get Date/Time In Seconds() -> (seconds since 1Jan1904=w293:timestamp)
    n254 = Format Date/Time String(time format string (%c)="%Y-%m-%d %H:%M:%S%2u", seconds (now)=w293) -> (date/time string=w289:string)  [unwired: 1 in]
    n255 = Build Array(w289, w292, w214, w273, w279, w256, w284, w280, w281, w264, w240, w206, w239, w238, w221, w218, w217) -> (w220:string[])
  }
  n256 = Unbundle(w80) -> (w79:bool, "VISA resource name out"=w78:refnum<visa-resource-name>, "error out"=w77:errorcluster)
  n257 = Unbundle(w85) -> (w84:bool, "VISA out"=w83:refnum<visa-resource-name>, "error out"=w82:errorcluster)
  n258 = Unbundle(w89) -> (w88:bool, "VISA resource name out"=w87:refnum<visa-resource-name>, "error out"=w86:errorcluster)
  n259 = case shown="True" w26 {
    tunnel: w25 -> [_ w691]
    tunnel: w24 -> [_ w690]
    frame False {
    }
    frame True {
      n260 = VISA Close(VISA resource name=w691, error in (no error)=w690) -> ()  [unwired: 1 out]
    }
  }
  n261 = Unbundle(w51) -> (w56:bool, "VISA resource name out"=w55:refnum<visa-resource-name>, "error out"=w54:errorcluster)
  n262 = case shown="True" w43 {
    tunnel: [w692 w712] -> w41
    tunnel: w44 -> [_ w711]
    tunnel: w45 -> [_ w710]
    tunnel: w47 -> [_ w706]
    tunnel: w46 -> [_ w705]
    tunnel: [w692 w704] -> w42
    tunnel: [w693 w701] -> w40
    tunnel: w38 -> [w693 w700]
    tunnel: w30 -> [_ w697]
    tunnel: [w692 w696] -> w33
    tunnel: w32 -> [_ w695]
    tunnel: w31 -> [_ w694]
    frame False {
      w692 = errorcluster {"status"=FALSE, "code"=0, "source"=""} ("error out")
    }
    frame True {
      n263 = call <vilib>:"DAQmx Stop Task.vi"("task/channels in"=w695, "error in"=w694) -> ("task out"=w698:refnum<k21>, "error out"=w699:errorcluster)  [unwired: 12 in]
      n264 = call <vilib>:"DAQmx Stop Task.vi"("task/channels in"=w706, "error in"=w705) -> ("task out"=w708:refnum<k21>, "error out"=w707:errorcluster)  [unwired: 12 in]
      n265 = call <vilib>:"DAQmx Stop Task.vi"("task/channels in"=w711, "error in"=w710) -> ("task out"=w709:refnum<k21>, "error out"=w713:errorcluster)  [unwired: 12 in]
      n266 = VISA Clear(VISA resource name=w697, error in (no error)=w700) -> (VISA resource name out=w703:refnum<visa-resource-name>, error out=w702:errorcluster)
      n267 = call <vilib>:"DAQmx Clear Task.vi"("task in"=w698, "error in"=w699) -> ("error out"=w696:errorcluster)  [unwired: 13 in]
      n268 = call <vilib>:"DAQmx Clear Task.vi"("task in"=w708, "error in"=w707) -> ("error out"=w704:errorcluster)  [unwired: 13 in]
      n269 = call <vilib>:"DAQmx Clear Task.vi"("task in"=w709, "error in"=w713) -> ("error out"=w712:errorcluster)  [unwired: 13 in]
      n270 = VISA Close(VISA resource name=w703, error in (no error)=w702) -> (error out=w701:errorcluster)
    }
  }
  n271 = case shown="True" w88 {
    tunnel: w87 -> [_ w717]
    tunnel: w86 -> [w714 w716]
    tunnel: [w714 w715] -> w90
    frame False {
    }
    frame True {
      n272 = call "Enable Output.vi"("error in (no error)"=w716, "Enable Output (T: Enable)"=FALSE, "VISA resource name"=w717) -> ("error out"=w718:errorcluster, "VISA resource name out"=w720:refnum<visa-resource-name>)  [unwired: 7 in]
      n273 = call "Close.vi"("error in (no error)"=w718, "VISA resource name"=w720) -> ("error out"=w715:errorcluster)  [unwired: 9 in]
    }
  }
  n274 = case shown="True" w56 {
    tunnel: w55 -> [_ w723]
    tunnel: w54 -> [w721 w722]
    tunnel: [w721 w724] -> w50
    frame False {
    }
    frame True {
      w727 = FALSE  # Output (F:Off)
      n275 = call "Enable Output.vi"("error in (no error)"=w722, "Enable Output (F:Off)"=w727, "VISA resource name"=w723) -> ("error out"=w725:errorcluster, "VISA resource name out"=w726:refnum<visa-resource-name>)  [unwired: 7 out]
      n276 = call "Close.vi"("error in (no error)"=w725, "VISA resource name"=w726) -> ("error out"=w724:errorcluster)  [unwired: 9 out]
    }
  }
  n277 = case shown="False" w84 {
    tunnel: w82 -> [w728 w731]
    tunnel: [w728 w730] -> w91
    tunnel: w83 -> [_ w729]
    frame False {
    }
    frame True {
      n278 = call "srsQcm200Close.vi"("error in"=w731, "Visa in"=w729) -> ("error out"=w730:errorcluster)  [unwired: 3 in]
    }
  }
  n279 = case shown="True" w79 {
    tunnel: w78 -> [_ w735]
    tunnel: w77 -> [w732 w734]
    tunnel: [w732 w733] -> w76
    frame False {
    }
    frame True {
      n280 = VISA Close(VISA resource name=w735, error in (no error)=w734) -> (error out=w733:errorcluster)
    }
  }
  n281 = Merge Errors(w33, w42, w41, w40) -> (w39:errorcluster)
  n282 = Merge Errors(w50, w76, w90, w91, w61, w39) -> (w98:errorcluster)
  n283 = call <vilib>:"Simple Error Handler.vi"("error in (no error)"=w98) -> ()  [unwired: 4 in, 5 out]
  n284 = Build Array("date/time", "min elapsed", "Keithley 6430 resistance (Ohm)", "J-KEM temp (C)", "Keithley 2420 resistance (Ohm)" ("element"), "QCM adsorbed mass (g)", "QCM freq (Hz)", "QCM resistance (Ohm)", "O2 partial pressure (Torr)" ("element"), "O2 concentration (PPM)" ("element"), "chamber pressure (Torr)" ("element"), "chamber RH (%)" ("element"), "gas flow (sccm)" ("element"), "vapor flow (sccm)" ("element"), "gas sensor" ("element"), "humidity (%)" ("element"), "temp (C)" ("element"), "Experiment Notes") -> (w68:string[])
  n285 = call-poly <vilib>:"Write To Spreadsheet File.vi"("1D data"=w68, "file path (dialog if empty)"=w60) -> ("new file path (Not A Path if cancelled)"=w69:path)  [unwired: 6 in]
  n286 = call-poly <vilib>:"Write To Spreadsheet File.vi"("append to file? (new file:F)"=TRUE, "2D data"=w97, "file path (dialog if empty)"=w69) -> ()  [unwired: 5 in, 1 out]
